vi "Initialize Default.vi"(8 "error in (no error)":errorcluster, 11 "Core Threads Configuration in":refnum<class "Core Thread Configuration.lvclass">) -> (0 "error out":errorcluster, 3 "Core Threads Configuration out":refnum<class "Core Thread Configuration.lvclass">)   [LabVIEW 2017, in "DSF Core.lvlib" / "Core Thread Configuration.lvclass"]
uses:
  Core Thread Configuration.lvclass
  Typedefs/DSF Core Thread Configuration.ctl
  Core Thread Configuration.lvclass/Core Thread Configuration.ctl
  DSF Core.lvlib
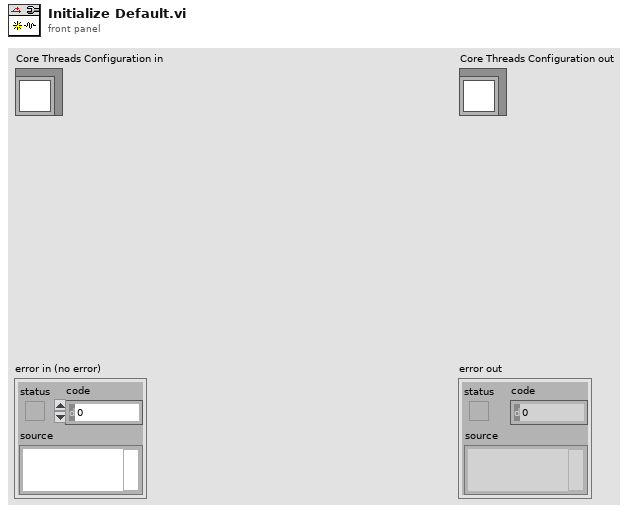
[diagram p1: front panel]
types:
  T1 = typedef "DSF Core.lvlib/DSF Core Thread Configuration.ctl" = cluster{"processor":i32, "priority offset":i16}
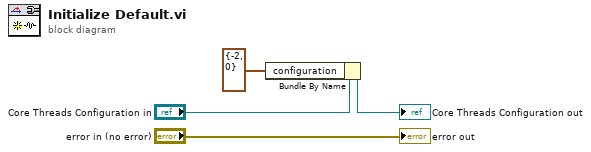
[diagram p0: block diagram]
diagram:
  n1 = Bundle By Name(cluster="Core Threads Configuration in", "configuration"=T1 {"processor"=-2, "priority offset"=0}) -> (→"Core Threads Configuration out":refnum<class "Core Thread Configuration.lvclass">)
  "error out" <- "error in (no error)"
